vi "ConvertLogDataToCSVString.vi"(9 "MFC Configuration":T1={"COM Port"=1, "Timeout (msec)"=100, "Setpoint"=0.0, "Valve State"=enum."Automatic", "Gas"=enum."Air", "Units"=enum."scc/m", "Serial Number"="", "Firmware Version"=""}, 10 "Heater Configuration":T5={"VISA Resource"="", "COM Port"=1, "Setpoint"=0.0, "Standby?"=FALSE}, 11 "Log Data":T6[](array[typedef])) -> (3 "CSV String":string)   [LabVIEW 2012]
uses:
  HardwareLogData.ctl
  HardwareDisplayData.ctl
  HeaterConfiguration.ctl
  MFCConfiguration.ctl
  libs/Sierra-M100/Public/Controls/ValveState.ctl
  libs/Sierra-M100/Public/Controls/Gas.ctl
  libs/Sierra-M100/Public/Controls/Units.ctl
  libs/Sierra-M100/Sierra-M100.lvlib
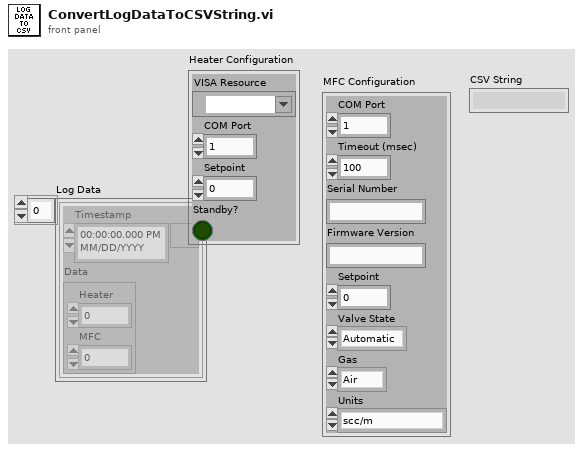
[diagram p1: front panel]
types:
  T1 = typedef "MFCConfiguration.ctl" = cluster{"COM Port":u32, "Timeout (msec)":u32, "Setpoint":dbl, "Valve State":T2, "Gas":T3, "Units":T4, "Serial Number":string, "Firmware Version":string}
  T2 = typedef "Sierra-M100.lvlib/ValveState.ctl" = enum16{"Automatic", "Closed", "Purge"}
  T3 = typedef "Sierra-M100.lvlib/Gas.ctl" = enum16{"Air", "Argon", "CO2", "CO", "Helium", "Hydrogen", "Methane", "Nitrogen", "Nitrous Oxide", "Oxygen"}
  T4 = typedef "Sierra-M100.lvlib/Units.ctl" = enum16{"scc/s", "scc/m", "scc/H", "Ncc/s", "Ncc/m", "Ncc/H", "SCF/s", "SCF/m", "SCF/H", "NM3/s", "NM3/m", "NM3/H", "SM3/s", "SM3/m", "SM3/H", "sl/s", "sl/m", "sl/H", "NL/s", "NL/m", "Nl/H", "g/s", "g/m", "g/H", "kg/s", "kg/m", "kg/H", "lb/s", "lb/m", "lb/H"}
  T5 = typedef "HeaterConfiguration.ctl" = cluster{"VISA Resource":refnum<visa-resource-name>, "COM Port":u8, "Setpoint":dbl, "Standby?":bool}
  T6 = typedef "HardwareLogData.ctl" = cluster{"Timestamp":timestamp, "Data":T7}
  T7 = typedef "HardwareDisplayData.ctl" = cluster{"Heater":dbl, "MFC":dbl}
  T8 = typedef "MFCDisplayValveState.ctl" = enum16{"Not Connected", "Automatic", "Closed", "Purge"}
  T9 = typedef "HeaterDisplayState.ctl" = enum16{"Not Connected", "Run", "Standby"}
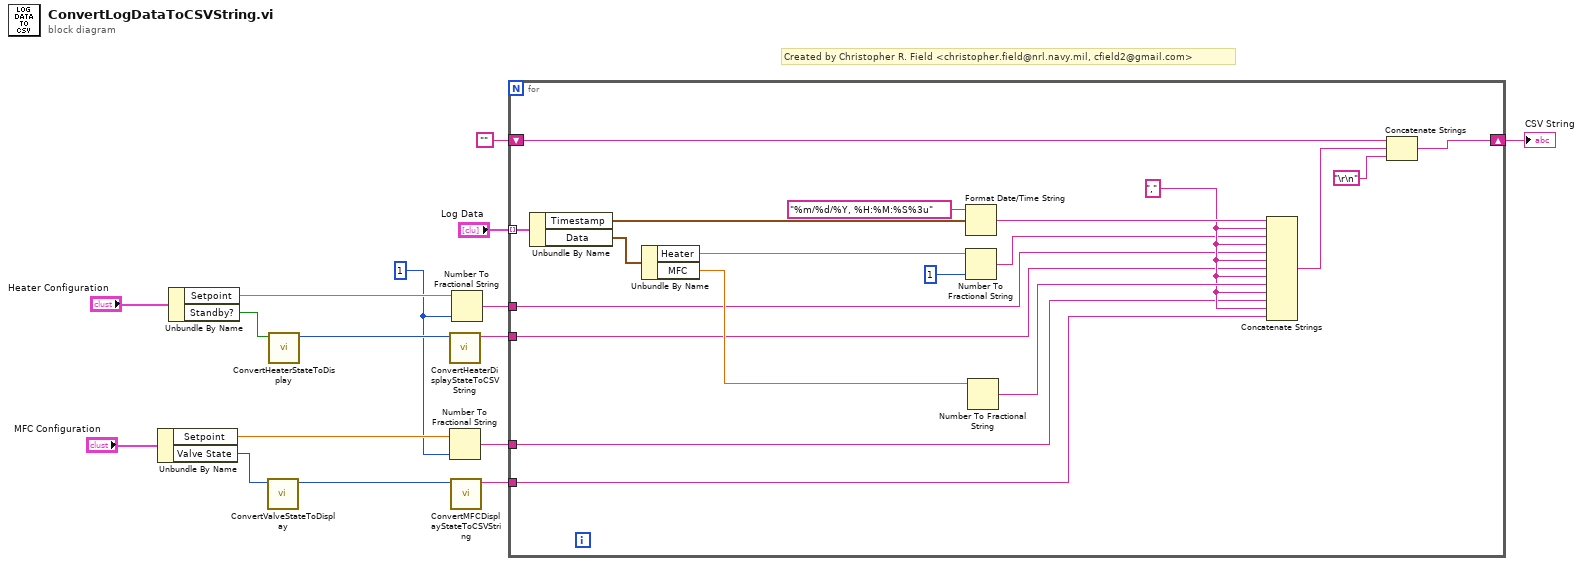
[diagram p0: block diagram]
diagram:
  w3 = i16 1 ("precision (6)")
  # "Created by Christopher R. Field <christopher.field@nrl.navy.mil, cfield2@gmail.com>"
  n1 = Unbundle By Name("MFC Configuration") -> ("Setpoint"=w4:dbl, "Valve State"=w11:T2)
  n2 = Unbundle By Name("Heater Configuration") -> ("Setpoint"=w9:dbl, "Standby?"=w10:bool)
  n3 = call "ConvertValveStateToDisplay.vi"("Valve State"=w11) -> ("MFC Valve State"=w2:T8)  [unwired: 10 in]
  n4 = call "ConvertHeaterStateToDisplay.vi"("Standby?"=w10) -> ("Heater Display State"=w7:T9)  [unwired: 10 in]
  n5 = call "ConvertHeaterDisplayStateToCSVString.vi"("Heater Display State"=w7) -> ("CSV String"=w6:string)  [unwired: 10 in]
  n6 = Number To Fractional String(number=w4, precision (6)=w3) -> (F-format string=w5:string)  [unwired: 2 in]
  n7 = call "ConvertMFCDisplayStateToCSVString.vi"("MFC Valve State"=w2) -> ("CSV String"=w1:string)  [unwired: 10 in]
  n8 = Number To Fractional String(number=w9, precision (6)=w3) -> (F-format string=w8:string)  [unwired: 2 in]
  n9 = for {
    tunnel: "Log Data" -> [w35] mode=indexing
    shift-right: [w26] -> w14
    shift-left: "" -> [w28]
    tunnel: w8 -> [w20]
    tunnel: w6 -> [w19]
    tunnel: w5 -> [w18]
    tunnel: w1 -> [w17]
    w29 = "," ("string")
    n10 = Unbundle By Name(w35) -> ("Timestamp"=w34:timestamp, "Data"=w24:T7)
    n11 = Unbundle By Name(w24) -> ("Heater"=w22:dbl, "MFC"=w21:dbl)
    n12 = Format Date/Time String(time format string (%c)="%m/%d/%Y, %H:%M:%S%3u", seconds (now)=w34) -> (date/time string=w32:string)  [unwired: 1 in]
    n13 = Number To Fractional String(number=w22, precision (6)=i16 1) -> (F-format string=w23:string)  [unwired: 2 in]
    n14 = Number To Fractional String(number=w21) -> (F-format string=w31:string)  [unwired: 3 in]
    n15 = Concatenate Strings(w32, w29, w23, w29, w20, w29, w19, w29, w31, w29, w18, w29, w17) -> (w27:string)
    n16 = Concatenate Strings(w28, w27, "\r\n") -> (w26:string)
  }
  "CSV String" <- w14
